vi "SpinnerExample.vi"() -> ()   [LabVIEW 2012]
uses:
  Control/Spinner.xctl
  Instance           1 22Saved   SpinnerExample .vi
panel:
  out "String":string="Instructions:\n\nThe rotation speed of the spinner is controlled by a time variable triangle function. See the left waveform graph. \n\nThe spinner rotates clockwise if the speed is positive. Otherwise, it rotates counterclockwise.\n\nNote click \"STOP\" or the Abort button to stop the VI. "
  out "Spinner":dbl(xcontrol)
  out "Rotation Speed of the Spinner":dynamicdata(graph)
  in  "stop":bool
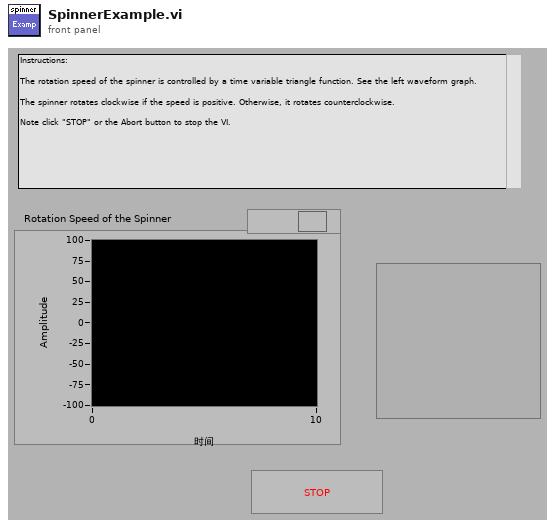
[diagram p1: front panel]
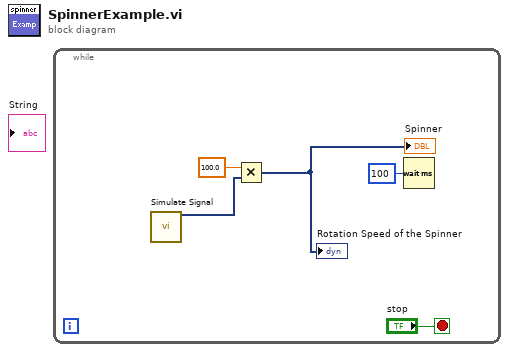
[diagram p0: block diagram]
diagram:
  n1 = while {
    stop <- "stop" stop-if-true
    n2 = call "Simulate Signal"() -> ("Triangle"=w3:dynamicdata)  [unwired: 14 in, 1 out]
    n3 = Multiply(x=100.0, y=w3) -> (x*y=→"Rotation Speed of the Spinner" →"Spinner":dynamicdata)
    n4 = Wait (ms)(milliseconds to wait=u32 100) -> ()  [unwired: 1 out]
  }
